vi "FTW-Test-JSON-Datatypes.vi"() -> ()   [LabVIEW 2013]
uses:
  source/JSON/FTW-JSON-Validate.vi
  source/Reflection/FTW-Reflection-Type.vi
  source/JSON/FTW-JSON-Native-GetFlattenedValue.vi
  source/CodeGen/JSON Deserialize/FTW-JSON-Deserialize.xnode
  source/JSON/FTW-JSON-Core-GetFlattenedValue.vi
  source/JSON/FTW-JSON-Core-LibraryFilepath.vi
  source/JSON/FTW-JSON-Core-LibraryError.vi
panel:
  out "Pass":bool
  out "error out":errorcluster
  out "element":T1 {"subobject"."EXT" format="%_32g"; "subobject"."DBL" format="%_32g"; "subobject"."SGL" format="%_32g"; "EXT" format="%_32g"; "DBL" format="%_32g"; "SGL" format="%_32g"}
  in  "Object":string="{\n  \"booleanfalse\": false,\n  \"booleantrue\": true,\n  \"U8\": 8,\n  \"U16\": 16,\n  \"U32\": 32,\n  \"U64\": 64,\n  \"I8\": -8,\n  \"I16\": -16,\n  \"I32\": -32,\n  \"I64\": -64,\n  \"SGL\": 1.23456789,\n  \"DBL\": 1.2345678901234567,\n  \"EXT\": 1.2345678901234567,\n  \"nullstring\": null,\n  \"stringempty\": \"\",\n  \"stringHW\": \"Hello World\",\n  \"EnumU8\": \"U8\",\n  \"EnumU16\": \"U16\",\n  \"EnumU32\": \"U32\",\n  \"Path\": \"c:\\\\some folder\\\\some file.txt\",\n  \"array\": [1,2,3],\n  \"visa resource\": \"myresource\",\n  \"VIrefnum\": \"0x123456789ABCDEF0\",\n  \"subobject\": {\n    \"booleanfalse\": false,\n    \"booleantrue\": true,\n    \"U8\": 8,\n    \"U16\": 16,\n    \"U32\": 32,\n    \"U64\": 64,\n    \"I8\": -8,\n    \"I16\": -16,\n    \"I32\": -32,\n    \"I64\": -64,\n    \"SGL\": 1.23456789,\n    \"DBL\": 1.2345678901234567,\n    \"EXT\": 1.2345678901234567,\n    \"nullstring\": null,\n    \"stringempty\": \"\",\n    \"stringHW\": \"Hello World\",\n    \"EnumU8\": \"U8\",\n    \"EnumU16\": \"U16\",\n    \"EnumU32\": \"U32\",\n    \"Path\": \"c:\\\\some folder\\\\some file.txt\",\n    \"array\": [4,5,6],\n    \"visa resource\": \"myresource\",\n    \"VIrefnum\": \"0x123456789ABCDEF0\"\n  },\n  \"unusedpair\": \"whatever\"\n}"
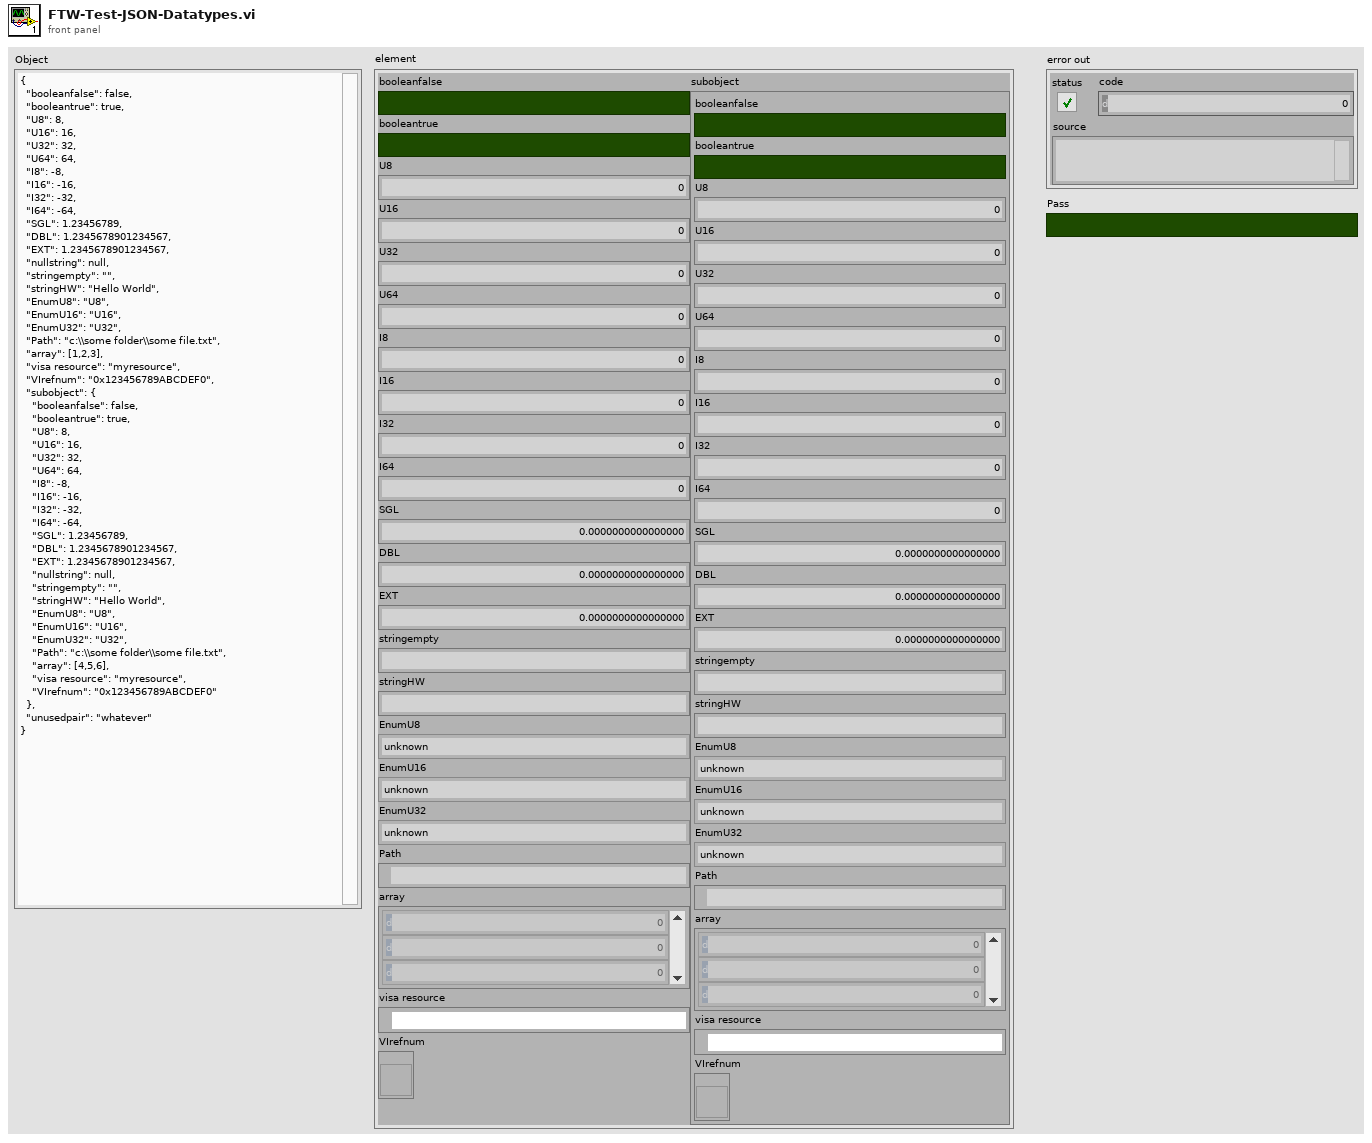
[diagram p1: front panel]
types:
  T1 = cluster{"booleanfalse":bool, "booleantrue":bool, "U8":u8, "U16":u16, "U32":u32, "U64":u64, "I8":i8, "I16":i16, "I32":i32, "I64":i64, "SGL":sgl, "DBL":dbl, "EXT":ext, "stringempty":string, "stringHW":string, "EnumU8":enum8{"unknown", "U8"}, "EnumU16":enum16{"unknown", "U16"}, "EnumU32":enum32{"unknown", "U32"}, "Path":path, "array":i32[], "visa resource":refnum<visa-resource-name>, "VIrefnum":refnum<vi>, "subobject":cluster{"booleanfalse":bool, "booleantrue":bool, "U8":u8, "U16":u16, "U32":u32, "U64":u64, "I8":i8, "I16":i16, "I32":i32, "I64":i64, "SGL":sgl, "DBL":dbl, "EXT":ext, "stringempty":string, "stringHW":string, "EnumU8":enum8{"unknown", "U8"}, "EnumU16":enum16{"unknown", "U16"}, "EnumU32":enum32{"unknown", "U32"}, "Path":path, "array":i32[], "visa resource":refnum<visa-resource-name>, "VIrefnum":refnum<vi>}}
  T2 = cluster{"booleanfalse":bool, "booleantrue":bool, "U8":u8, "U16":u16, "U32":u32, "U64":u64, "I8":i8, "I16":i16, "I32":i32, "I64":i64, "SGL":sgl, "DBL":dbl, "EXT":ext, "stringempty":string, "stringHW":string, "EnumU8":enum8{"unknown", "U8"}, "EnumU16":enum16{"unknown", "U16"}, "EnumU32":enum32{"unknown", "U32"}, "Path":path, "array":i32[], "visa resource":refnum<visa-resource-name>, "VIrefnum":refnum<vi>}
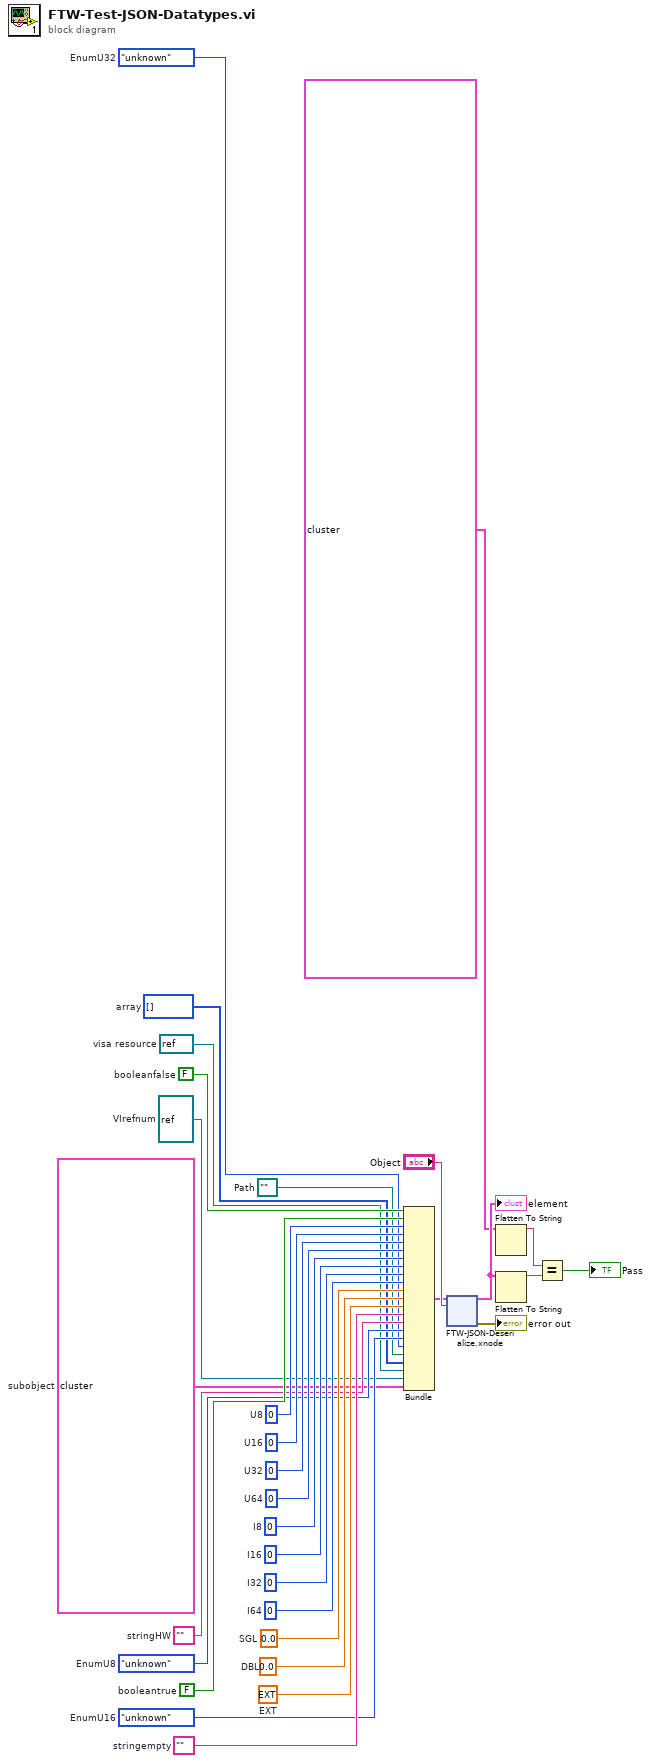
[diagram p0: block diagram]
diagram:
  w1 = refnum<vi> refnum  # VIrefnum
  w7 = refnum<visa-resource-name> refnum  # visa resource
  w8 = i32[] []  # array
  w9 = path ""  # Path
  w10 = T2 {"booleanfalse"=FALSE, "booleantrue"=FALSE, "U8"=0, "U16"=0, "U32"=0, "U64"=0, "I8"=0, "I16"=0, "I32"=0, "I64"=0, "SGL"=0.0, "DBL"=0.0, "EXT"=0.0, "stringempty"="", "stringHW"="", "EnumU8"=enum."unknown", "EnumU16"=enum."unknown", "EnumU32"=enum."unknown", "Path"=path "", "array"=[], "visa resource"="", "VIrefnum"=refnum}  # subobject
  w11 = enum32{"unknown", "U32"}."unknown"  # EnumU32
  w12 = enum16{"unknown", "U16"}."unknown"  # EnumU16
  w13 = enum8{"unknown", "U8"}."unknown"  # EnumU8
  w14 = ""  # stringHW
  w15 = ""  # stringempty
  w17 = FALSE  # booleantrue
  w18 = FALSE  # booleanfalse
  w19 = ext 0.0  # EXT
  w20 = 0.0  # DBL
  w21 = sgl 0.0  # SGL
  w22 = i64 0  # I64
  w23 = 0  # I32
  w24 = i16 0  # I16
  w25 = i8 0  # I8
  w26 = u64 0  # U64
  w27 = u32 0  # U32
  w28 = u16 0  # U16
  w29 = u8 0  # U8
  n1 = Bundle("booleanfalse"=w18, "booleantrue"=w17, "U8"=w29, "U16"=w28, "U32"=w27, "U64"=w26, "I8"=w25, "I16"=w24, "I32"=w23, "I64"=w22, "SGL"=w21, "DBL"=w20, "EXT"=w19, "stringempty"=w15, "stringHW"=w14, "EnumU8"=w13, "EnumU16"=w12, "EnumU32"=w11, "Path"=w9, "array"=w8, "visa resource"=w7, "VIrefnum"=w1, "subobject"=w10) -> (w16:T1)  [unwired: 1 in]
  n2 = xnode "FTW-JSON-Deserialize.xnode"("Type and Defaults"=w16, "JSON String"="Object") -> ("Values"=w5:T1, "error out"=→"error out":errorcluster)  [unwired: 1 in]
  "element" <- w5
  n3 = Flatten To String(anything=T1 {"booleanfalse"=FALSE, "booleantrue"=TRUE, "U8"=8, "U16"=16, "U32"=32, "U64"=64, "I8"=-8, "I16"=-16, "I32"=-32, "I64"=-64, "SGL"=1.2345679, "DBL"=1.2345678901234567, "EXT"=1.2345678901234567, "stringempty"="", "stringHW"="Hello World", "EnumU8"=enum."U8", "EnumU16"=enum."U16", "EnumU32"=enum."U32", "Path"=path "c:/some folder/some file.txt", "array"=[1, 2, 3], "visa resource"="myresource", "VIrefnum"=refnum, "subobject"={"booleanfalse"=FALSE, "booleantrue"=TRUE, "U8"=8, "U16"=16, "U32"=32, "U64"=64, "I8"=-8, "I16"=-16, "I32"=-32, "I64"=-64, "SGL"=1.2345679, "DBL"=1.2345678901234567, "EXT"=1.2345678901234567, "stringempty"="", "stringHW"="Hello World", "EnumU8"=enum."U8", "EnumU16"=enum."U16", "EnumU32"=enum."U32", "Path"=path "c:/some folder/some file.txt", "array"=[4, 5, 6], "visa resource"="myresource", "VIrefnum"=refnum}} ("element")) -> (data string=w6:string)  [unwired: 3 in, 2 out]
  n4 = Flatten To String(anything=w5) -> (data string=w4:string)  [unwired: 3 in, 2 out]
  n5 = Equal?(x=w6, y=w4) -> (x = y?=→"Pass":bool)
